vi "CreateLoopArray.vi"(8 "Randomize":bool, 9 "Loop Stepsize":dbl=1.0, 10 "Loop End":dbl, 11 "Loop Start":dbl) -> (3 "Loop Array":dbl[](array[numeric]))   [LabVIEW 2015]
uses:
  <vilib>/Analysis/1siggen.llb/Riffle Array (DBL).vi
  <vilib>/Analysis/NI_AALBase.lvlib
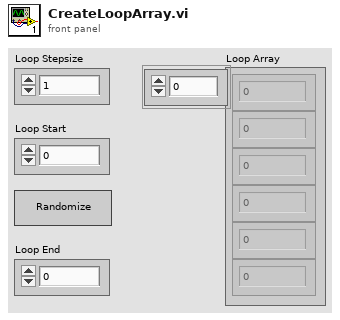
[diagram p1: front panel]
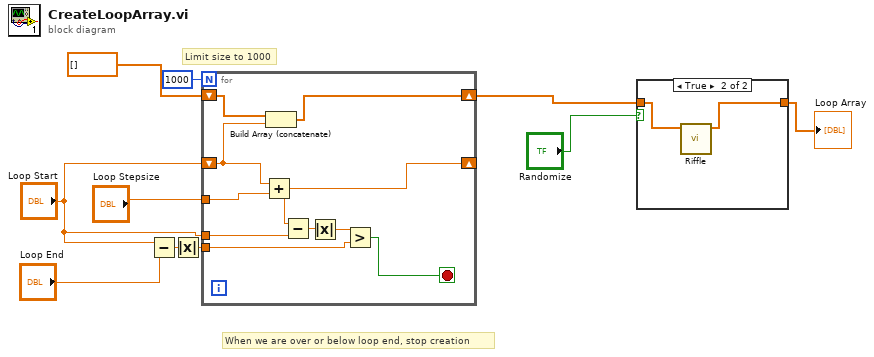
[diagram p0: block diagram]
diagram:
  # "When we are over or below loop end, stop creation"
  # "Limit size to 1000"
  n1 = Subtract(x="Loop Start", y="Loop End") -> (x-y=w4:dbl)
  n2 = Absolute Value(x=w4) -> (abs(x)=w6:dbl)
  n3 = for {
    N: 1000 -> [_]
    shift-right: [w17] -> w8
    shift-left: dbl[] [] -> [w20]
    shift-right: [w15] -> _
    shift-left: "Loop Start" -> [w18]
    tunnel: "Loop Stepsize" -> [w19]
    tunnel: "Loop Start" -> [w14]
    tunnel: w6 -> [w12]
    stop <- w11 stop-if-true
    n4 = Add(x=w18, y=w19) -> (x+y=w15:dbl)
    n5 = Build Array (concatenate)(w20, w18) -> (w17:dbl[])
    n6 = Subtract(x=w15, y=w14) -> (x-y=w16:dbl)
    n7 = Absolute Value(x=w16) -> (abs(x)=w13:dbl)
    n8 = Greater?(x=w13, y=w12) -> (0:w11:bool)
  }
  n9 = case shown="True" "Randomize" {
    tunnel: w8 -> [w21 w23]
    tunnel: [w21 w22] -> w9
    frame False {
    }
    frame True {
      n10 = call-poly <vilib>:"Riffle.vi"("X"=w23) -> ("Riffled {X}"=w22:dbl[])  [unwired: 8 in, 2 out]
    }
  }
  "Loop Array" <- w9
